vi "Handle LogRec.vi"(8 "error in":errorcluster, 10 "LogRecord":refnum<class "LogRecord.lvclass">, 11 "FileHandler in":refnum<class "RotateFileHandler.lvclass">) -> (0 "error out":errorcluster, 3 "FileHandler out":refnum<class "RotateFileHandler.lvclass">)   [LabVIEW 2024, in "RotateFileHandler.lvclass"]
uses:
  RotateFileHandler.lvclass
  <vilib>/Hampel Software Engineering/HSE Logger/LogRecord/LogRecord.lvclass
  RotateFileHandler.lvclass/RotateFileHandler.ctl
  LogRotation/LogRotationHandler.lvclass
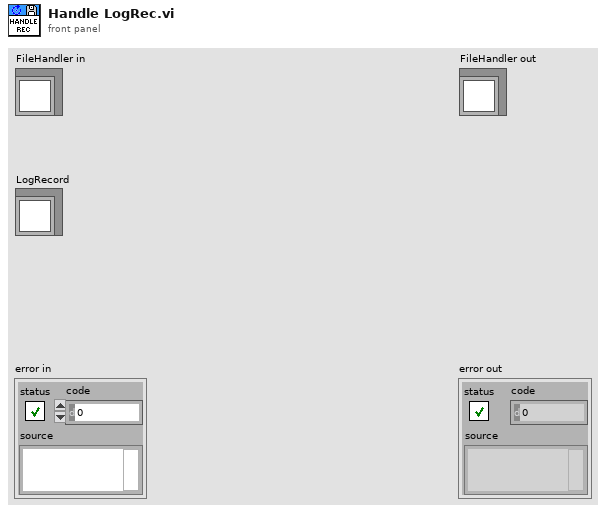
[diagram p1: front panel]
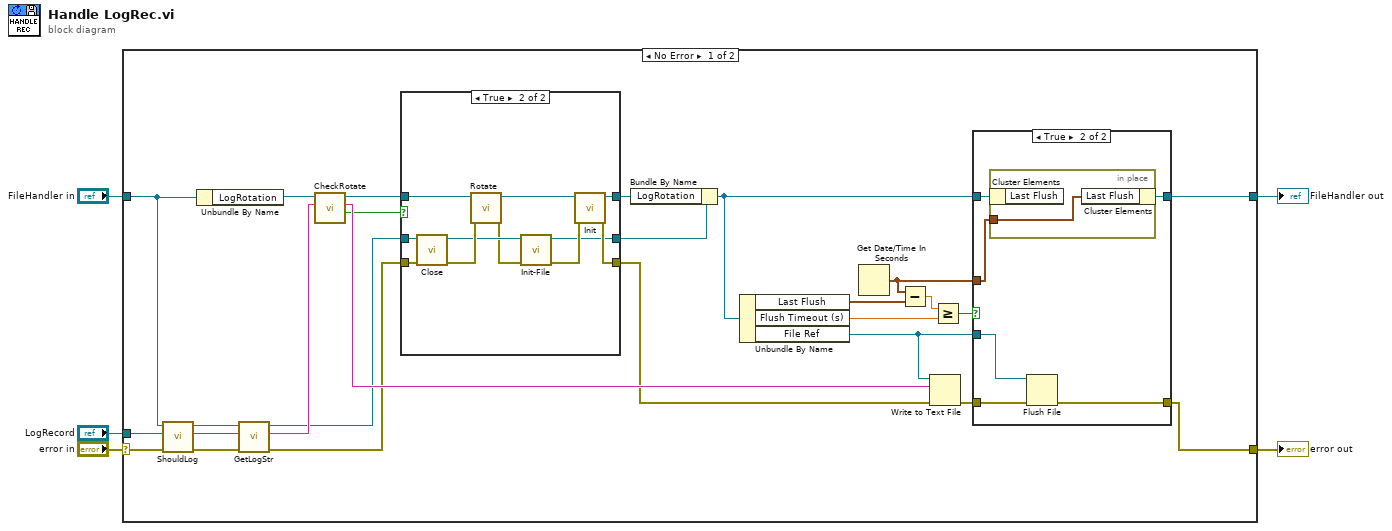
[diagram p0: block diagram]
diagram:
  n1 = case shown="No Error" "error in" {
    selector: "error in" -> [w31 w56]
    tunnel: [w26 w56] -> w4
    tunnel: [w23 w55] -> w2
    tunnel: "FileHandler in" -> [w17 w55]
    tunnel: "LogRecord" -> [w30 _]
    frame No Error {
      n2 = call "ShouldLog.vi"("error in (no error)"=w31, "LogRecord"=w30, "FileHandler in"=w17) -> ("error out"=w28:errorcluster, "LogRecord out"=w29:refnum<class "LogRecord.lvclass">, "FileHandler out"=w22:refnum<class "RotateFileHandler.lvclass">)  [unwired: 5 in, 1 out]
      n3 = Unbundle By Name(w17) -> ("LogRotation"=w16:refnum<class "LogRotationHandler.lvclass">)
      n4 = call "GetLogStr.vi"("error in (no error)"=w28, "LogRecord in"=w29, "FileHandler in"=w22) -> ("error out"=w11:errorcluster, "LogLine"=w15:string, "FileHandler out"=w9:refnum<class "RotateFileHandler.lvclass">)  [unwired: 6 in]
      n5 = call "CheckRotate.vi"("To Log in"=w15, "LogRotationHandler in"=w16) -> ("Rotate?"=w12:bool, "To Log out"=w14:string, "LogRotationHandler out"=w13:refnum<class "LogRotationHandler.lvclass">)  [unwired: 7 in]
      n6 = case shown="True" w12 {
        tunnel: w13 -> [w41 w54]
        tunnel: w9 -> [w43 w53]
        tunnel: w11 -> [w42 w52]
        tunnel: [w42 w48] -> w10
        tunnel: [w43 w44] -> w8
        tunnel: [w41 w49] -> w6
        frame False {
        }
        frame True {
          n7 = call-dynamic "Close.vi"("error in"=w52, "FileHandler in"=w53) -> ("error out"=w51:errorcluster, "FileHandler out"=w47:refnum<class "RotateFileHandler.lvclass">)  [unwired: 8 in]
          n8 = call "Rotate.vi"("error in (no error)"=w51, "LogRotationHandler in"=w54) -> ("error out"=w46:errorcluster, "LogRotationHandler out"=w50:refnum<class "LogRotationHandler.lvclass">)  [unwired: 8 in]
          n9 = call "Init-File.vi"("error in (no error)"=w46, "FileHandler in"=w47) -> ("error out"=w45:errorcluster, "FileHandler out"=w44:refnum<class "RotateFileHandler.lvclass">)  [unwired: 8 in]
          n10 = call "Init.vi"("error in (no error)"=w45, "LogRotationHandler in"=w50) -> ("error out"=w48:errorcluster, "LogRotationHandler out"=w49:refnum<class "LogRotationHandler.lvclass">)  [unwired: 8 in]
        }
      }
      n11 = Bundle By Name(cluster=w8, "LogRotation"=w6) -> (w7:refnum<class "RotateFileHandler.lvclass">)
      n12 = Unbundle By Name(w7) -> ("Last Flush"=w25:timestamp, "Flush Timeout (s)"=w24:dbl, "File Ref"=w27:refnum<file>)
      n13 = Get Date/Time In Seconds() -> (seconds since 1Jan1904=w19:timestamp)
      n14 = Subtract(x=w19, y=w25) -> (x-y=w21:dbl)
      n15 = Write to Text File(file (use dialog)=w27, text=w14, error in=w10) -> (error out=w18:errorcluster)  [unwired: 1 in, 2 out]
      n16 = Greater Or Equal?(x=w21, y=w24) -> (x >= y?=w20:bool)
      n17 = case shown="True" w20 {
        tunnel: w18 -> [w32 w39]
        tunnel: w27 -> [_ w38]
        tunnel: w19 -> [_ w34]
        tunnel: w7 -> [w33 w36]
        tunnel: [w33 w35] -> w23
        tunnel: [w32 w37] -> w26
        frame False {
        }
        frame True {
          n18 = in-place {
            in-place-border: w34 -> [w40]
            n19 = in-place-cluster #1(w36) -> ()  [unwired: 1 out]
            n20 = in-place-cluster #1("Last Flush"=w40) -> (w35:refnum<class "RotateFileHandler.lvclass">)
          }
          n21 = Flush File(refnum=w38, error in=w39) -> (error out=w37:errorcluster)  [unwired: 1 out]
        }
      }
    }
    frame Error {
    }
  }
  "error out" <- w4
  "FileHandler out" <- w2
